vi "PinholesSingle.vi"(4 "Current Threshold [nA]":dbl, 5 "Probe Card Channels":i32=32, 6 "Channel":i32, 7 "Measurement Parameters":T1) -> (0 "Compliance?":bool, 1 "channel excluded":bool, 2 "Current [nA]":dbl, 3 "Flag":i32)   [LabVIEW 2013]
panel:
  out "DAQ complete?":bool
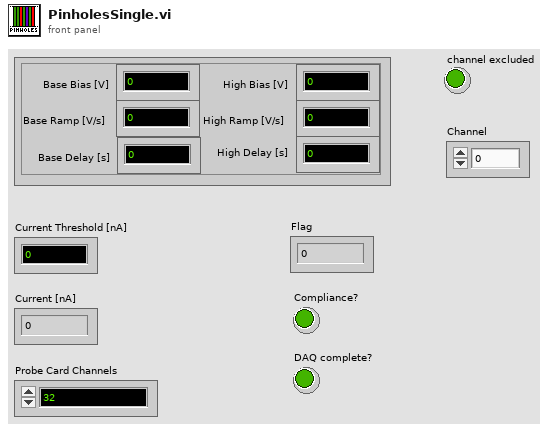
[diagram p1: front panel]
types:
  T1 = cluster{"Base Bias [V]":dbl, "Base Ramp [V/s]":dbl, "High Bias [V]":dbl, "High Ramp [V/s]":dbl, "High Delay [s]":i32, "Base Delay [s]":i32}
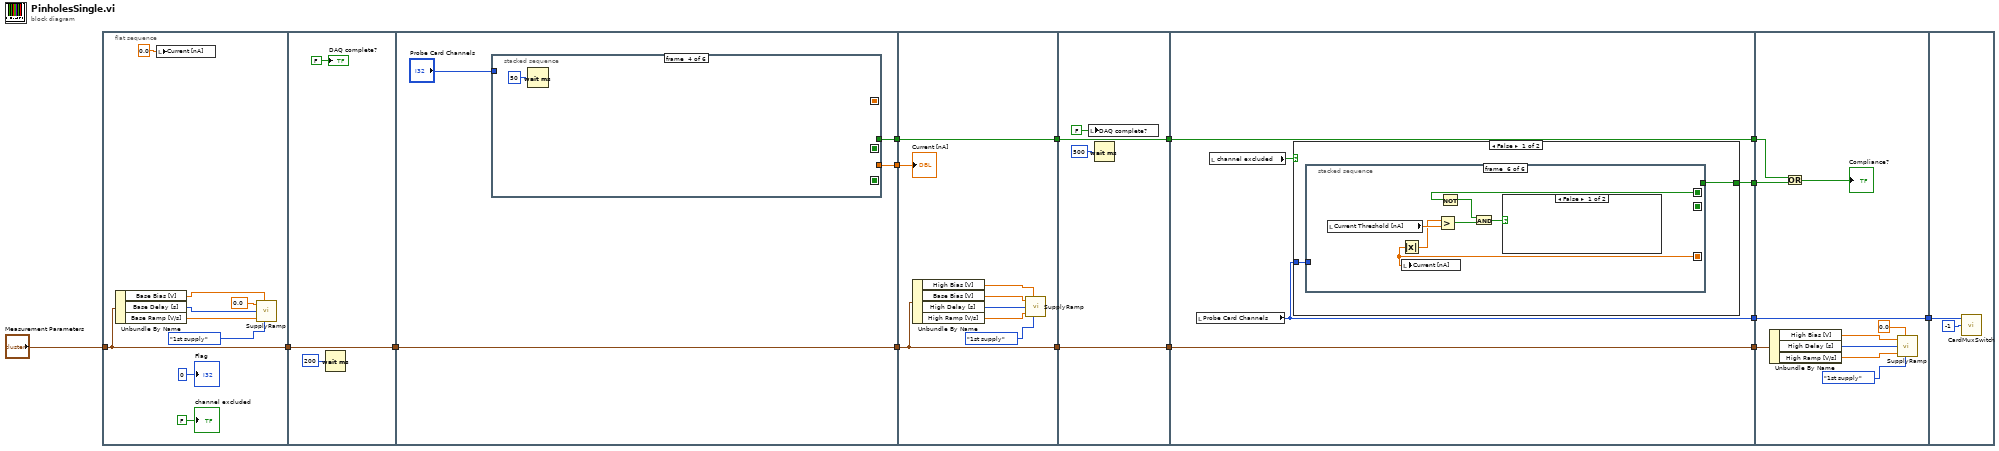
[diagram p0: block diagram]
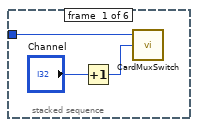
[diagram p2: hidden frame]
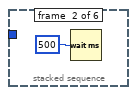
[diagram p3: hidden frame]
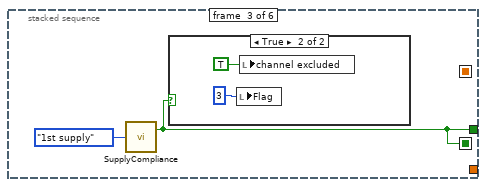
[diagram p4: hidden frame]
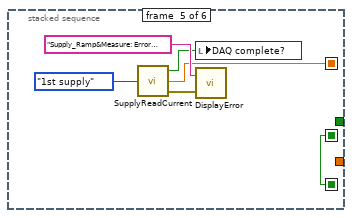
[diagram p6: hidden frame]
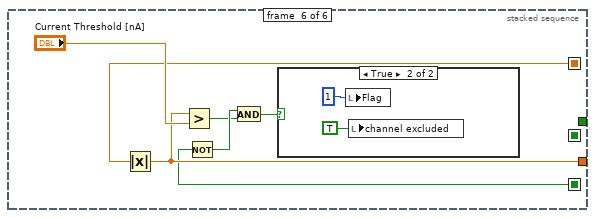
[diagram p7: hidden frame]
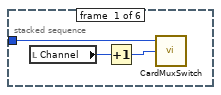
[diagram p9: hidden frame]
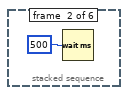
[diagram p10: hidden frame]
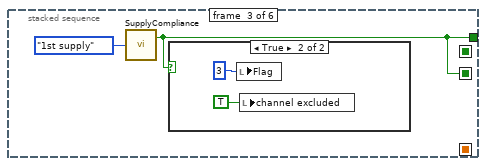
[diagram p11: hidden frame]
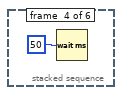
[diagram p13: hidden frame]
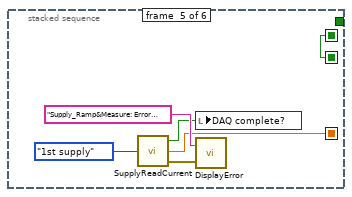
[diagram p14: hidden frame]
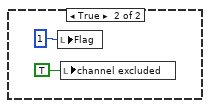
[diagram p15: hidden frame]
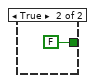
[diagram p16: hidden frame]
diagram:
  n1 = flat-sequence {
    tunnel: "Measurement Parameters" -> [w16]
    tunnel: [w16] -> w14
    tunnel: w14 -> [w26]
    tunnel: [w26] -> w13
    tunnel: w13 -> [w31]
    tunnel: [w31] -> w12
    tunnel: [w30] -> w11
    tunnel: [w29] -> w10
    tunnel: w12 -> [w58]
    tunnel: [w58] -> w9
    tunnel: w11 -> [w60]
    tunnel: w10 -> [w61]
    tunnel: [w61] -> w8
    tunnel: w9 -> [w67]
    tunnel: [w67] -> w7
    tunnel: w8 -> [w66]
    tunnel: [w66] -> w5
    tunnel: w7 -> [w72]
    tunnel: [w72] -> w6
    tunnel: w5 -> [w71]
    tunnel: [w71] -> w4
    tunnel: [w70] -> w3
    tunnel: [w68] -> w2
    tunnel: w6 -> [w106]
    tunnel: w4 -> [w104]
    tunnel: w3 -> [w103]
    tunnel: w2 -> [w102]
    tunnel: [w102] -> w1
    tunnel: w1 -> [w110]
    frame #0 {
      n2 = Unbundle By Name(w16) -> ("Base Bias [V]"=w23:dbl, "Base Delay [s]"=w22:i32, "Base Ramp [V/s]"=w21:dbl)
      n3 = local write "Current [nA]"(0.0) -> ()
      n4 = call "SupplyRamp.vi"("Starting Voltage"=0.0, "Requested Voltage"=w23, "Step Delay"=w22, "Step Size"=w21, "1st/2nd Supply"=enum16{"1st supply", "2nd supply"}."1st supply") -> ()  [unwired: 3 in, 3 out]
      "Flag" <- 0
      "channel excluded" <- FALSE
    }
    frame #1 {
      n5 = Wait (ms)(milliseconds to wait=200) -> ()  [unwired: 1 out]
      "DAQ complete?" <- FALSE
    }
    frame #2 {
      n6 = stacked-sequence {
        seq-local: [_ _ w37 _ _ _] -> [_ _ _ _ w42 _]
        seq-local: [_ _ _ _ w43 _] -> [_ _ _ _ _ w49]
        seq-local: [_ _ _ _ w42 _] -> [_ _ _ _ _ w47]
        tunnel: "Probe Card Channels" -> [w34 _ _ _ _ _]
        tunnel: [_ _ w37 _ _ _] -> w29
        tunnel: [_ _ _ _ _ w48] -> w30
        frame #0 {
          n7 = Increment(x="Channel") -> (x+1=w33:i32)
          n8 = call "CardMuxSwitch.vi"("No. of probe channels"=w34, "switch to channel"=w33) -> ()  [unwired: 2 in, 3 out]
        }
        frame #1 {
          n9 = Wait (ms)(milliseconds to wait=500) -> ()  [unwired: 1 out]
        }
        frame #2 {
          n10 = call "SupplyCompliance.vi"("1st/2nd Supply"=enum16{"1st supply", "2nd supply"}."1st supply") -> ("Compliance exceeded?"=w37:bool)  [unwired: 2 in, 1 out]
          n11 = case shown="True" w37 {
            frame False {
            }
            frame True {
              n12 = local write "Flag"(3) -> ()
              n13 = local write "channel excluded"(TRUE) -> ()
            }
          }
        }
        frame #3 {
          n14 = Wait (ms)(milliseconds to wait=50) -> ()  [unwired: 1 out]
        }
        frame #4 {
          n15 = call "SupplyReadCurrent.vi"("1st/2nd Supply"=enum16{"1st supply", "2nd supply"}."1st supply") -> ("Error Out"=w45:errorcluster, "Current [nA]"=w43:dbl, "Done!"=w44:bool)  [unwired: 2 in]
          n16 = local write "DAQ complete?"(w44) -> ()
          n17 = call "DisplayError.vi"("Error In"=w45, "Error String In"="Supply_Ramp&Measure: Error reading data" ("Error String IN")) -> ()
        }
        frame #5 {
          n18 = Absolute Value(x=w49) -> (abs(x)=w48:dbl)
          n19 = Greater?(x=w48, y="Current Threshold [nA]") -> (0:w50:bool)
          n20 = Not(x=w47) -> (.not. x?=w52:bool)
          n21 = And(x=w52, y=w50) -> (x .and. y?=w51:bool)
          n22 = case shown="True" w51 {
            frame False {
            }
            frame True {
              n23 = local write "Flag"(1) -> ()
              n24 = local write "channel excluded"(TRUE) -> ()
            }
          }
        }
      }
    }
    frame #3 {
      n25 = Unbundle By Name(w58) -> ("High Bias [V]"=w57:dbl, "Base Bias [V]"=w56:dbl, "High Delay [s]"=w63:i32, "High Ramp [V/s]"=w62:dbl)
      n26 = call "SupplyRamp.vi"("Starting Voltage"=w56, "Requested Voltage"=w57, "Step Delay"=w63, "Step Size"=w62, "1st/2nd Supply"=enum16{"1st supply", "2nd supply"}."1st supply") -> ()  [unwired: 3 in, 3 out]
      "Current [nA]" <- w60
    }
    frame #4 {
      n27 = local write "DAQ complete?"(FALSE) -> ()
      n28 = Wait (ms)(milliseconds to wait=500) -> ()  [unwired: 1 out]
    }
    frame #5 {
      n29 = local read "Probe Card Channels"() -> (w68:i32)
      n30 = local read "channel excluded"() -> (w69:bool)
      n31 = case shown="False" w69 {
        tunnel: w68 -> [w74 _]
        tunnel: [w73 FALSE] -> w70
        frame False {
          n32 = stacked-sequence {
            seq-local: [_ _ w80 _ _ _] -> [_ _ _ _ w85 _]
            seq-local: [_ _ _ _ w86 _] -> [_ _ _ _ _ w90]
            seq-local: [_ _ _ _ w85 _] -> [_ _ _ _ _ w91]
            tunnel: w74 -> [w76 _ _ _ _ _]
            tunnel: [_ _ w80 _ _ _] -> w73
            frame #0 {
              n33 = local read "Channel"() -> (w75:i32)
              n34 = Increment(x=w75) -> (x+1=w77:i32)
              n35 = call "CardMuxSwitch.vi"("No. of probe channels"=w76, "switch to channel"=w77) -> ()  [unwired: 2 in, 3 out]
            }
            frame #1 {
              n36 = Wait (ms)(milliseconds to wait=500) -> ()  [unwired: 1 out]
            }
            frame #2 {
              n37 = call "SupplyCompliance.vi"("1st/2nd Supply"=enum16{"1st supply", "2nd supply"}."1st supply") -> ("Compliance exceeded?"=w80:bool)  [unwired: 2 in, 1 out]
              n38 = case shown="True" w80 {
                frame False {
                }
                frame True {
                  n39 = local write "Flag"(3) -> ()
                  n40 = local write "channel excluded"(TRUE) -> ()
                }
              }
            }
            frame #3 {
              n41 = Wait (ms)(milliseconds to wait=50) -> ()  [unwired: 1 out]
            }
            frame #4 {
              n42 = call "SupplyReadCurrent.vi"("1st/2nd Supply"=enum16{"1st supply", "2nd supply"}."1st supply") -> ("Error Out"=w88:errorcluster, "Current [nA]"=w86:dbl, "Done!"=w87:bool)  [unwired: 2 in]
              n43 = local write "DAQ complete?"(w87) -> ()
              n44 = call "DisplayError.vi"("Error In"=w88, "Error String In"="Supply_Ramp&Measure: Error reading data" ("Error String IN")) -> ()
            }
            frame #5 {
              n45 = local read "Current Threshold [nA]"() -> (w93:dbl)
              n46 = Absolute Value(x=w90) -> (abs(x)=w92:dbl)
              n47 = local write "Current [nA]"(w90) -> ()
              n48 = Greater?(x=w92, y=w93) -> (0:w94:bool)
              n49 = Not(x=w91) -> (.not. x?=w96:bool)
              n50 = And(x=w96, y=w94) -> (x .and. y?=w95:bool)
              n51 = case shown="False" w95 {
                frame False {
                }
                frame True {
                  n52 = local write "Flag"(1) -> ()
                  n53 = local write "channel excluded"(TRUE) -> ()
                }
              }
            }
          }
        }
        frame True {
        }
      }
    }
    frame #6 {
      n54 = Unbundle By Name(w106) -> ("High Bias [V]"=w100:dbl, "High Delay [s]"=w108:i32, "High Ramp [V/s]"=w107:dbl)
      n55 = Or(x=w104, y=w103) -> (x .or. y?=→"Compliance?":bool)
      n56 = call "SupplyRamp.vi"("Starting Voltage"=w100, "Requested Voltage"=0.0, "Step Delay"=w108, "Step Size"=w107, "1st/2nd Supply"=enum16{"1st supply", "2nd supply"}."1st supply") -> ()  [unwired: 3 in, 3 out]
    }
    frame #7 {
      n57 = call "CardMuxSwitch.vi"("No. of probe channels"=w110, "switch to channel"=-1) -> ()  [unwired: 2 in, 3 out]
    }
  }
